vi "Read_PCE.vi"(8 "error in":errorcluster, 11 "VISA resource name":refnum<visa-resource-name>) -> (0 "error out":errorcluster, 3 "Chaîne":string)   [LabVIEW 2011]
panel:
  out "return count":u32
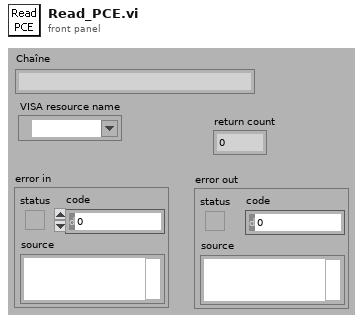
[diagram p1: front panel]
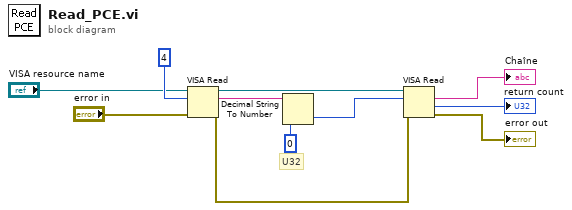
[diagram p0: block diagram]
diagram:
  # "U32"
  n1 = VISA Read(VISA resource name="VISA resource name", byte count=u32 4 ("requested byte count"), error in (no error)="error in") -> (VISA resource name out=w6:refnum<visa-resource-name>, read buffer=w9:string, error out=w1:errorcluster)  [unwired: 1 out]
  n2 = Decimal String To Number(string=w9, default (0L)=u32 0 ("default (0 I32)")) -> (number=w10:u32)  [unwired: 1 in, 1 out]
  n3 = VISA Read(VISA resource name=w6, byte count=w10, error in (no error)=w1) -> (read buffer=→"Chaîne":string, return count=→"return count":u32, error out=→"error out":errorcluster)  [unwired: 1 out]
